vi "parseTemperature.vi"(8 "error in (no error)":errorcluster, 10 "response":string, 11 "PlainTextResponseParser in":refnum<class "PlainTextResponseParser.lvclass">) -> (0 "error out":errorcluster, 2 "temperature":i32, 3 "PlainTextResponseParser out":refnum<class "PlainTextResponseParser.lvclass">)   [LabVIEW 2023, in "AbstractFactory.lvlib" / "PlainTextResponseParser.lvclass"]
uses:
  PlainTextResponseParser.lvclass
  PlainTextResponseParser.lvclass/PlainTextResponseParser.ctl
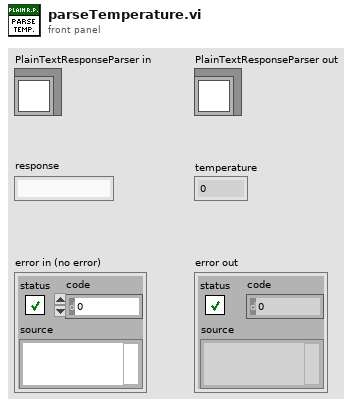
[diagram p1: front panel]
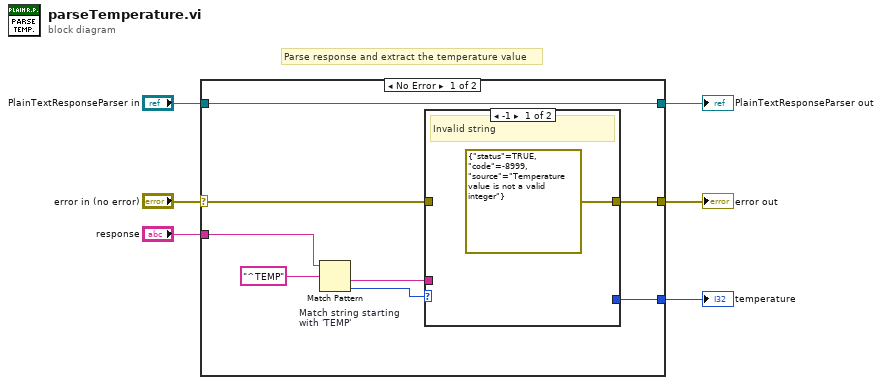
[diagram p0: block diagram]
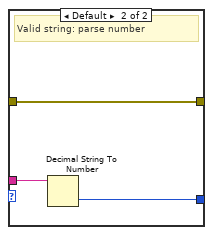
[diagram p2: hidden frame]
diagram:
  # "Parse response and extract the temperature value"
  n1 = case shown="No Error" "error in (no error)" {
    selector: "error in (no error)" -> [w12 w20]
    tunnel: [w11 w20] -> w5
    tunnel: [w9 _] -> w4
    tunnel: [w8 w19] -> w2
    tunnel: "PlainTextResponseParser in" -> [w8 w19]
    tunnel: "response" -> [w7 _]
    frame No Error {
      n2 = Match Pattern "Match string starting with 'TEMP'"(string=w7, regular expression="^TEMP") -> (after substring=w10:string, offset past match=w13:i32)  [unwired: 1 in, 2 out]
      n3 = case shown="-1" w13 {
        tunnel: w12 -> [_ w16]
        tunnel: [errorcluster {"status"=TRUE, "code"=-8999, "source"="Temperature value is not a valid integer"} ("error in (no error)") w16] -> w11
        tunnel: w10 -> [_ w18]
        tunnel: [_ w17] -> w9
        frame -1 {
          # "Invalid string"
        }
        frame Default {
          # "Valid string: parse number"
          n4 = Decimal String To Number(string=w18) -> (number=w17:i32)  [unwired: 2 in, 1 out]
        }
      }
    }
    frame Error {
    }
  }
  "error out" <- w5
  "PlainTextResponseParser out" <- w2
  "temperature" <- w4
